vi "E443X_ESG_VSG_Configure_Frequency.vi"(0 "VISA Resource Name":refnum<visa-resource-name>, 1 "Freq Offset (0.0)":dbl format="%#_3g", 2 "Freq Multiplier (1.0)":dbl=1.0, 3 "Adjust Phase (0.0)":dbl format="%.3f", 5 "Frequency (1000.0)":dbl=1000.0 format="%#.3g", 7 "Freq Ref Set (0.0)":dbl format="%.8f", 9 "Freq Ref (T:ON)":bool=TRUE, 11 "error in (no error)":errorcluster {"code" format="%.0x"}, 12 "OptPhNoise (F:MD2 > 10khzOffset)":bool, 13 "Freq Mode (T:CW)":bool=TRUE) -> (4 "VISA Resource Name Out":refnum<visa-resource-name>, 15 "error out":errorcluster {"code" format="%.0x"})   [LabVIEW 2015]
doc: "This VI is used to set the modulation controls and the parameters associated with the carrier signal frequency.\n\nNotes:\nThis VI is used with ESG-A and ESG-D Series instruments only."
panel:
  # "MODE 1 < 10khz Offset"
  # "MODE 2 >10khz Offset"
  # "ON"
  # "OFF"
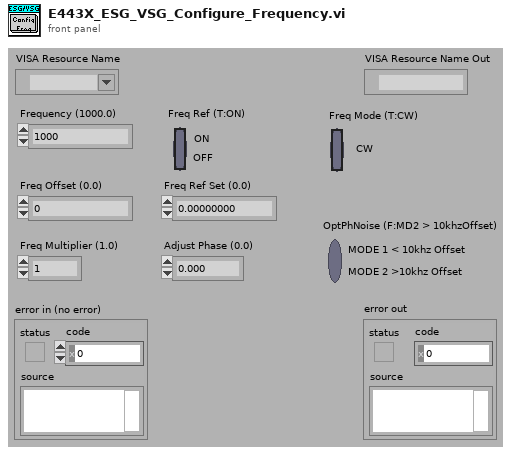
[diagram p1: front panel]
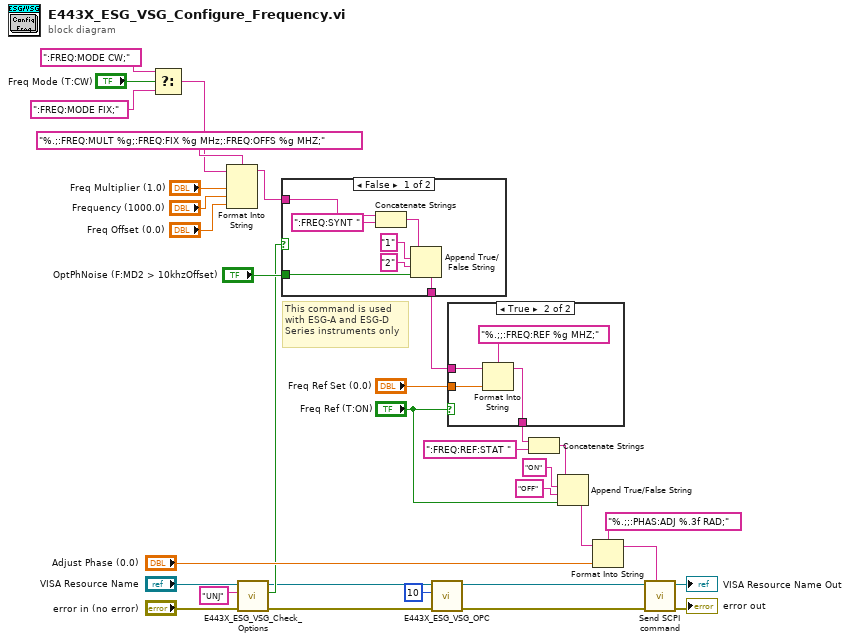
[diagram p0: block diagram]
diagram:
  # "This command is used \nwith ESG-A and ESG-D \nSeries instruments only"
  n1 = Select(t=":FREQ:MODE CW;", s="Freq Mode (T:CW)", f=":FREQ:MODE FIX;") -> (s? t:f=w1:string)
  n2 = Format Into String(format string="%.;:FREQ:MULT %g;:FREQ:FIX %g MHz;:FREQ:OFFS %g MHZ;", initial string=w1, "Freq Multiplier (1.0)", "Frequency (1000.0)", "Freq Offset (0.0)") -> (resulting string=w17:string)  [unwired: 1 in, 1 out]
  n3 = call "E443X_ESG_VSG_Check_Options.vi"("error in (no error)"="error in (no error)", "Search Options"="UNJ", "VISA Resource Name"="VISA Resource Name") -> ("error out"=w9:errorcluster, "Found"=w13:bool, "VISA Resource Name Out"=w8:refnum<visa-resource-name>)  [unwired: 6 in]
  n4 = case shown="False" w13 {
    tunnel: w17 -> [w36 w41]
    tunnel: "OptPhNoise (F:MD2 > 10khzOffset)" -> [w35 _]
    tunnel: [w34 w41] -> w16
    frame False {
      n5 = Concatenate Strings(w36, ":FREQ:SYNT ") -> (w39:string)
      n6 = Append True/False String(1:w35, 2:"2" ("false string"), 3:"1" ("true string"), 4:w39) -> (0:w34:string)
    }
    frame True {
    }
  }
  n7 = call "E443X_ESG_VSG_OPC.vi"("error in (no error)"=w9, "Wait (1000ms)"=u32 10, "VISA resource name"=w8) -> ("error out"=w6:errorcluster, "VISA resource name out"=w7:refnum<visa-resource-name>)  [unwired: 7 in]
  n8 = case shown="True" "Freq Ref (T:ON)" {
    tunnel: [w42 w43] -> w15
    tunnel: "Freq Ref Set (0.0)" -> [_ w46]
    tunnel: w16 -> [w42 w44]
    frame False {
    }
    frame True {
      n9 = Format Into String(format string="%.;;:FREQ:REF %g MHZ;", initial string=w44, w46) -> (resulting string=w43:string)  [unwired: 1 in, 1 out]
    }
  }
  n10 = Concatenate Strings(w15, ":FREQ:REF:STAT ") -> (w30:string)
  n11 = Append True/False String(1:"Freq Ref (T:ON)", 2:"OFF" ("false string"), 3:"ON" ("true string"), 4:w30) -> (0:w11:string)
  n12 = Format Into String(format string="%.;;:PHAS:ADJ %.3f RAD;", initial string=w11, "Adjust Phase (0.0)") -> (resulting string=w10:string)  [unwired: 1 in, 1 out]
  n13 = call "Send SCPI command.vi"("Send SCPI Command"=w10, "error in (no error)"=w6, "VISA resource name"=w7) -> ("error out"=→"error out":errorcluster, "VISA resource name out"=→"VISA Resource Name Out":refnum<visa-resource-name>)  [unwired: 7 in]
